vi "isConnected.vi"(8 "error in (no error)":errorcluster, 11 "Connection in":refnum<class "Connection.lvclass">) -> (0 "error out":errorcluster, 2 "connected":bool, 3 "Connection out":refnum<class "Connection.lvclass">)   [LabVIEW 2013, in "MQTT_Connection.lvlib" / "Connection.lvclass"]
uses:
  Connection.lvclass
  Connection.lvclass/Connection.ctl
  <vilib>/Utility/error.llb/Error Cluster From Error Code.vi
  <vilib>/ErrorRing/Error Ring.xnode
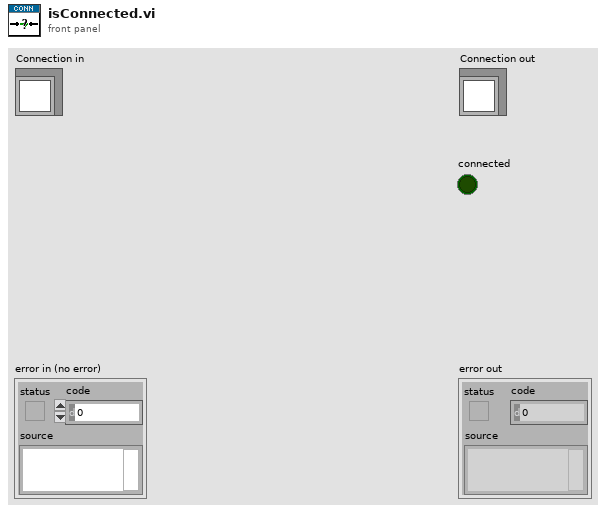
[diagram p1: front panel]
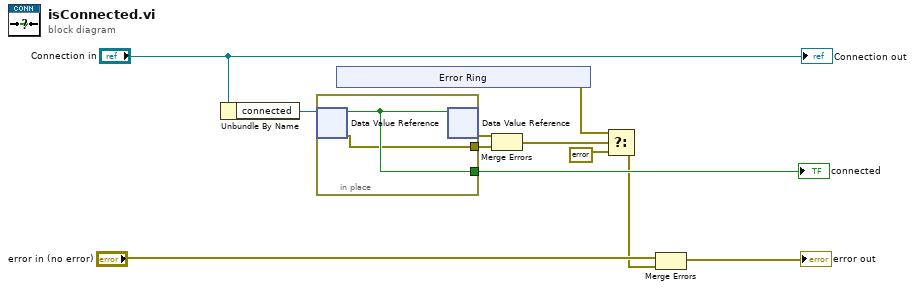
[diagram p0: block diagram]
diagram:
  n1 = Unbundle By Name("Connection in") -> ("connected"=w10:refnum<data-value>)
  n2 = in-place {
    in-place-border: [w13] -> w9
    in-place-border: [w12] -> w6
    n3 = in-place-dvr #1(w10) -> (w13:bool, w12:errorcluster)
    n4 = in-place-dvr #1(w13) -> (w5:errorcluster)  [unwired: 1 out]
  }
  "connected" <- w9
  n5 = xnode "Error Ring"() -> ("error out"=w2:errorcluster)
  n6 = Merge Errors(w5, w6) -> (w4:errorcluster)
  n7 = Select(t=w2, s=w4, f=errorcluster {"status"=FALSE, "code"=0, "source"=""} ("error out")) -> (s? t:f=w1:errorcluster)
  n8 = Merge Errors("error in (no error)", w1) -> (→"error out":errorcluster)
  "Connection out" <- "Connection in"
